vi "Worked Example--Chamber Conditions Cluster.vi"() -> ()   [LabVIEW 8.6]
uses:
  Instance           2 50Saved   Worked Example--Chamber Conditions Cluster .vi
panel:
  in  "stop":bool
  out "Chamber Conditions":T1={"Temperature (ºC)"=27.090074303959042, "Relative Humidity (%)"=65.79323643827468, "Pressure (mbar)"=1022.2555275919851} {"Relative Humidity (%)" scale=0.0..100.0; "Pressure (mbar)" scale=600.0..1100.0; "Temperature (ºC)" scale=20.0..30.0}
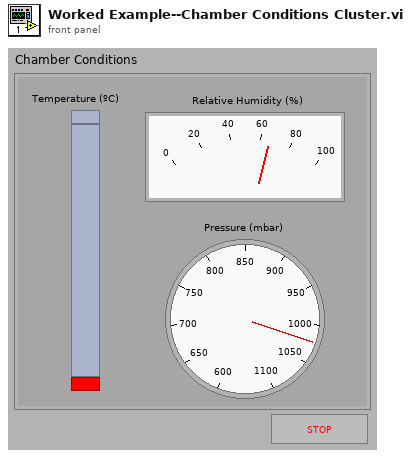
[diagram p1: front panel]
types:
  T1 = cluster{"Temperature (ºC)":dbl, "Relative Humidity (%)":dbl, "Pressure (mbar)":dbl}
  T2 = cluster{"Temp.":dbl, "Humidity":dbl, "Pressure":dbl}
  T3 = cluster{"T Voltage":dbl, "RH Voltage":dbl, "P Voltage":dbl}
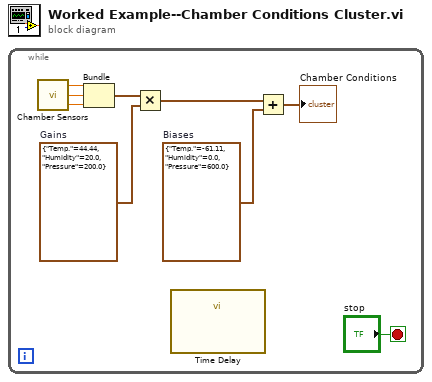
[diagram p0: block diagram]
diagram:
  n1 = while {
    stop <- "stop" stop-if-true
    w9 = T2 {"Temp."=44.44, "Humidity"=20.0, "Pressure"=200.0}  # Gains
    w7 = T2 {"Temp."=-61.11, "Humidity"=0.0, "Pressure"=600.0}  # Biases
    n2 = call "Chamber Sensors.vi"() -> ("P Voltage"=w2:dbl, "RH Voltage"=w3:dbl, "T Voltage"=w4:dbl)  [unwired: 3 in]
    n3 = Bundle("T Voltage"=w4, "RH Voltage"=w3, "P Voltage"=w2) -> (w1:T3)  [unwired: 1 in]
    n4 = Multiply(x=w1, y=w9) -> (x*y=w8:cluster{dbl, dbl, dbl})
    n5 = call "Time Delay"() -> ()  [unwired: 11 in, 1 out]
    n6 = Add(x=w8, y=w7) -> (x+y=→"Chamber Conditions":cluster{dbl, dbl, dbl})
  }
